vi "Map to Dictionary.vi"(8 "error in (no error)":errorcluster, 11 "map":T1) -> (0 "error out":errorcluster, 3 "Data (Dictionary)":T2[](array[typedef]))   [LabVIEW 2019, in "LV-Data.lvclass"]
uses:
  LV-Data.lvclass
  Typedefs/Dictionary--cluster.ctl
  Typedefs/Map Variant--map.ctl
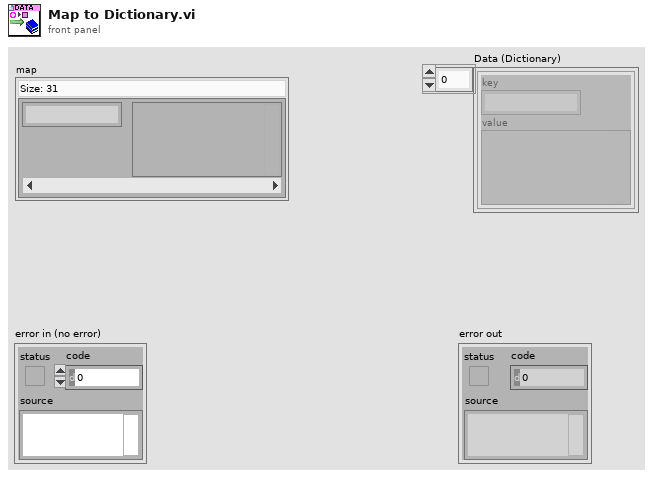
[diagram p1: front panel]
types:
  T1 = typedef "LV-Data.lvclass/Map Variant--map.ctl" = map{string, variant}
  T2 = typedef "LV-Data.lvclass/Dictionary--cluster.ctl" = cluster{"key":string, "value":variant}
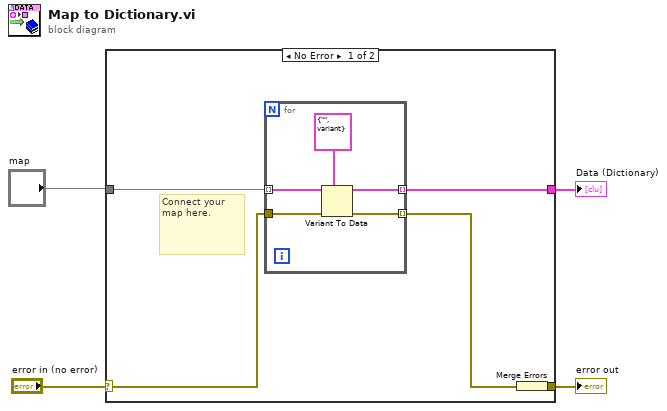
[diagram p0: block diagram]
diagram:
  n1 = case shown="No Error" "error in (no error)" {
    selector: "error in (no error)" -> [w8 w15]
    tunnel: [w6 w15] -> w4
    tunnel: "map" -> [w9 _]
    tunnel: [w5 _] -> w1
    frame No Error {
      # "Connect your map here."
      n2 = for {
        tunnel: w9 -> [w14] mode=indexing
        tunnel: w8 -> [w12]
        tunnel: [w11] -> w7 mode=indexing
        tunnel: [w10] -> w5 mode=indexing
        n3 = Variant To Data(error in=w12, type=T2 {"key"="", "value"=variant} ("key-value"), Variant=w14) -> (data=w10:T2, error out=w11:errorcluster)
      }
      n4 = Merge Errors(w7) -> (w6:errorcluster)
    }
    frame Error {
    }
  }
  "error out" <- w4
  "Data (Dictionary)" <- w1
